vi "Stop Core.vi"(10 "final error code":i32, 11 "Parent in":refnum<class "Message_Distributor_Class.lvclass">) -> (3 "Parent out":refnum<class "Message_Distributor_Class.lvclass">)   [LabVIEW 2023, in "Actor_Message_Distributor.lvlib" / "Message_Distributor_Class.lvclass"]
doc: "(<B>Filename</B>: Actor Framework.lvlib:Actor.lvclass:Stop Core.vi)\n\nDefines what the actor does before it stops. Use the <B>final error code</B> input to determine whether the actor shut down in response to an error.\n\nBy default, this method passes the Stop message along to all auto-stop nested actors. A descendant class may override this method to define additional behavior, such as shutting down any processes the actor initiated in its override of the Actor Core method."
uses:
  Message_Distributor_Class.lvclass
  Abstraction_Interface_Class/Abstraction_Interface_Class.lvclass
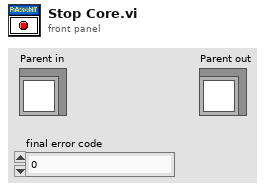
[diagram p1: front panel]
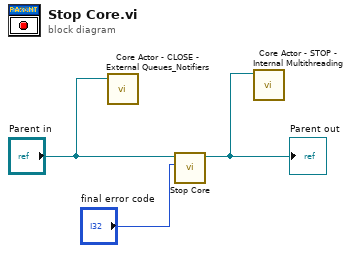
[diagram p0: block diagram]
diagram:
  n1 = call-dynamic "Core Actor - CLOSE - External Queues_Notifiers.vi"("Parent_Class in"="Parent in") -> ()  [unwired: 9 in, 2 out]
  n2 = call-parent "Stop Core.vi"("final error code"="final error code", "Actor in"="Parent in") -> ("Actor out"=w1:refnum<class "Message_Distributor_Class.lvclass">)  [unwired: 9 in]
  "Parent out" <- w1
  n3 = call-dynamic "Core Actor - STOP - Internal Multithreading.vi"("Parent_Class in"=w1) -> ()  [unwired: 9 in, 2 out]
